vi "ELVIS III v1.0 AI Continuous Config Bank A.vi"(0 "AI (Continuous) Channels FPGA Reference":T1, 1 "Bank Config":u8[](array[numeric]), 2 "Count (tick/s)":u32, 3 "error in (no error)":errorcluster) -> (10 "error out":errorcluster)   [LabVIEW 2021]
uses:
  <vilib>/myRIO/Common/Instrument Driver Framework/ELVIS III v1.0/AI Block/typedefs/ELVIS III AI Block Channels FPGA Reference.ctl
  <vilib>/rvi/errors/niLvFpgaAdjustHostInterfaceError.vi
  <vilib>/rvi/interface/nirviReadWriteControl/nirviReadWriteControl.xnode
  <vilib>/rvi/interface/Simulation/niFpgaSimulationCallBeginRW.vi
  NiFpgaLv.dll
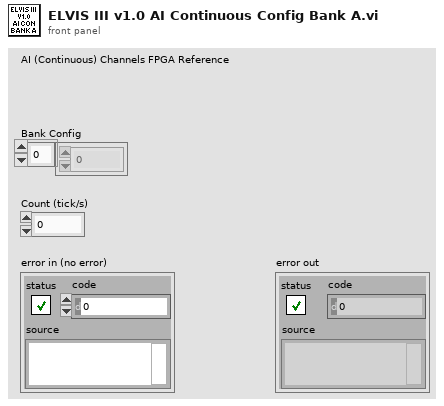
[diagram p1: front panel]
types:
  T1 = typedef "ELVIS III AI Block Channels FPGA Reference.ctl" = refnum<k20>
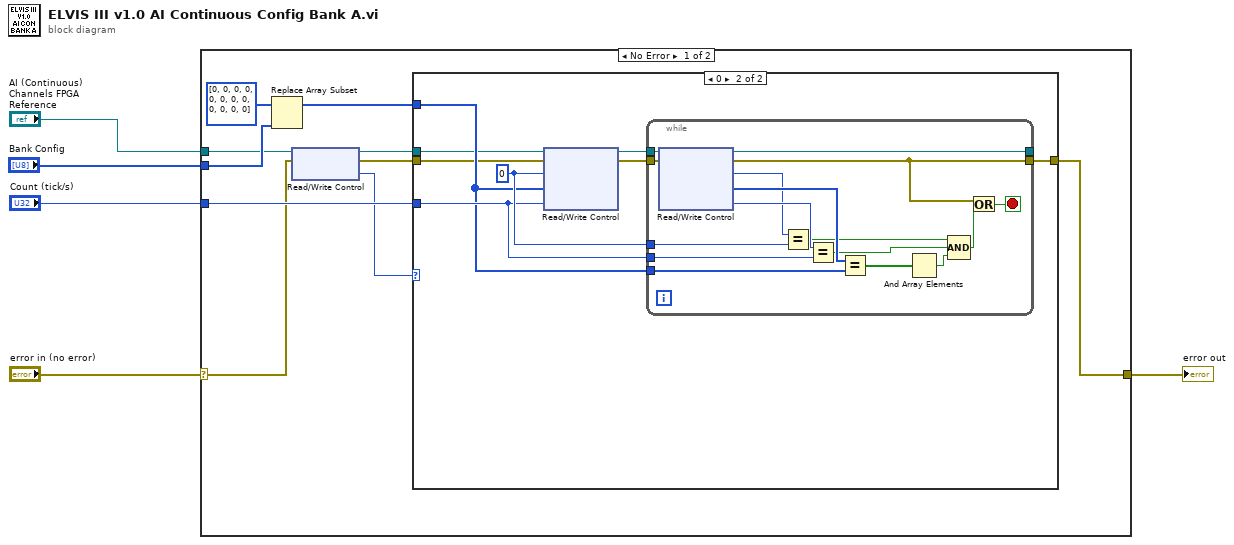
[diagram p0: block diagram]
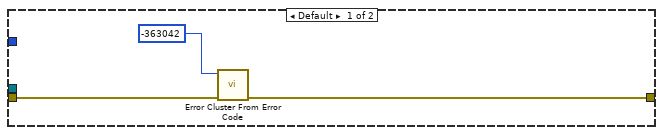
[diagram p2: hidden frame]
diagram:
  n1 = case shown="No Error" "error in (no error)" {
    selector: "error in (no error)" -> [w7 w43]
    tunnel: "AI (Continuous) Channels FPGA Reference" -> [w10 _]
    tunnel: "Count (tick/s)" -> [w12 _]
    tunnel: "Bank Config" -> [w13 _]
    tunnel: [w15 w43] -> w1
    frame No Error {
      n2 = Replace Array Subset(array=u8[] [0, 0, 0, 0, 0, 0, 0, 0, 0, 0, 0, 0] ("AI.A.CNFG"), new element=w13) -> (w11:u8[])  [unwired: 1 in]
      n3 = xnode "Read/Write Control"("FPGA VI Reference In"=w10, "error in"=w7) -> ("FPGA VI Reference Out"=w9:T1, "error out"=w6:errorcluster, "AI.A.CNT"=w8:u8)
      n4 = case shown="0" w8 {
        tunnel: [w16 w24] -> w15
        tunnel: w12 -> [_ w22]
        tunnel: w11 -> [_ w21]
        tunnel: w9 -> [_ w20]
        tunnel: w6 -> [w17 w19]
        frame Default {
          n5 = call <vilib>:"Error Cluster From Error Code.vi"("error in (no error)"=w17, "error code (0)"=-363042) -> ("error out"=w16:errorcluster)  [unwired: 7 in]
        }
        frame 0 {
          w23 = u8 0 ("AI.A.CNT")
          n6 = xnode "Read/Write Control"("FPGA VI Reference In"=w20, "error in"=w19, "AI.A.CNT"=w23, "AI.A.CNFG"=w21, "AI.A.CNTR"=w22) -> ("FPGA VI Reference Out"=w25:T1, "error out"=w26:errorcluster)
          n7 = while {
            tunnel: w25 -> [w42]
            tunnel: w26 -> [w41]
            tunnel: [w40] -> _
            tunnel: [w32] -> w24
            tunnel: w21 -> [w30]
            tunnel: w22 -> [w38]
            tunnel: w23 -> [w36]
            stop <- w31 stop-if-true
            n8 = xnode "Read/Write Control"("FPGA VI Reference In"=w42, "error in"=w41) -> ("FPGA VI Reference Out"=w40:T1, "error out"=w32:errorcluster, "AI.A.CNT"=w28:u8, "AI.A.CNFG"=w39:u8[], "AI.A.CNTR"=w37:u32)
            n9 = Equal?(x=w28, y=w36) -> (x = y?=w35:bool)
            n10 = Equal?(x=w37, y=w38) -> (x = y?=w34:bool)
            n11 = Equal?(x=w39, y=w30) -> (x = y?=w27:bool[])
            n12 = And Array Elements(Boolean array=w27) -> (logical AND=w29:bool)
            n13 = Compound Arithmetic op=AND(w35, w34, w29) -> (w33:bool)
            n14 = Or(x=w32, y=w33) -> (x .or. y?=w31:bool)
          }
        }
      }
    }
    frame Error {
    }
  }
  "error out" <- w1
